vi "Extract Complementary Image ROI.vi"(8 "error in (no error)":errorcluster, 10 "Image Model":T2, 11 "ROI in":T1 {"Contours"."Type" items=["No Selection", "Point", "Line", "Rectangle", "Oval", "Polygon", "Freehand Region", "Annulus", "Unused2", "Unused3", "Broken Line", "Freehand Line", "Rotated Rectangle"]}) -> (0 "error out":errorcluster, 3 "Complementary ROI":T1 {"Contours"."Type" items=["No Selection", "Point", "Line", "Rectangle", "Oval", "Polygon", "Freehand Region", "Annulus", "Unused2", "Unused3", "Broken Line", "Freehand Line", "Rotated Rectangle"]})   [LabVIEW 2021, in "Image.lvlib"]
doc: "Builds complementary ROI."
uses:
  Image.lvlib
  <vilib>/vision/Image Controls.llb/IMAQ Image.ctl
  <vilib>/vision/NI_Vision_Development_Module.lvlib
  Error/Error.lvlib
panel:
  # "see the AlliGator License on the block diagram (Ctrl+E or Window:Show Block Diagram)"
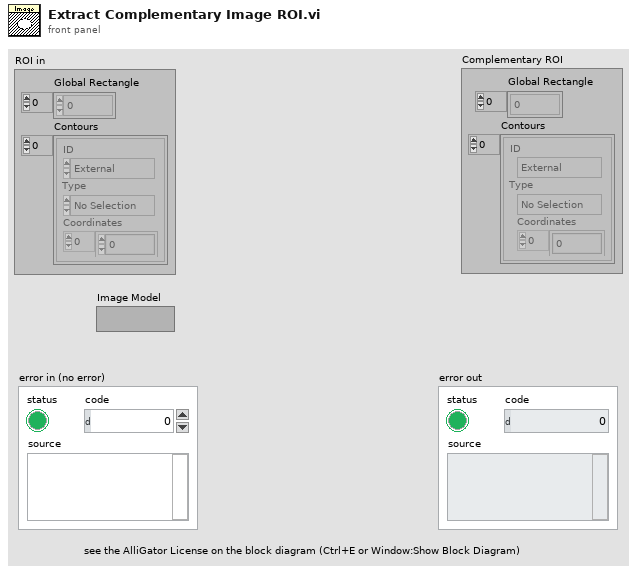
[diagram p1: front panel]
types:
  T1 = typedef "ROI Descriptor" = cluster{"Global Rectangle":i32[], "Contours":cluster{"ID":enum32{"External", "Internal"}, "Type":u32, "Coordinates":i32[]}[]}
  T2 = typedef "IMAQ Image.ctl" = refnum<image>
  T3 = typedef "Image Type" = u32
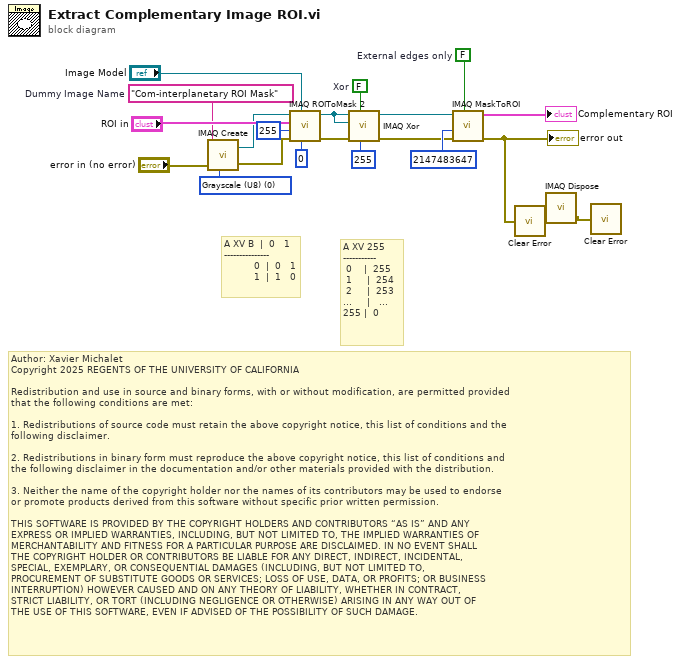
[diagram p0: block diagram]
diagram:
  w3 = FALSE  # Xor
  w11 = "Com-interplanetary ROI Mask"  # Dummy Image Name
  w12 = T3 0 items=["Grayscale (U8)", "Grayscale (I16)", "Grayscale (SGL)", "Complex (CSG)", "RGB (U32)", "HSL (U32)", "RGB (U64)", "Grayscale (U16)"] ("Image Type")
  w13 = FALSE  # External edges only
  # "Author: Xavier Michalet\nCopyright 2025 REGENTS OF THE UNIVERSITY OF CALIFORNIA\n\nRedistribution and use in source and binary forms, with or without modification, are permitted provided\nthat the following conditions are met:\n\n1. Redistributions of source code must retain the above copyright notice, this list of conditions and the\nfollowing disclaimer.\n\n2. Redistributions in binary form must reproduce the above copyright notice, this list of conditions and\nthe following disclaimer in the documentation and/or other materials provided with the distribution.\n\n3. Neither the name of the copyright holder nor the names of its contributors may be used to endorse \nor promote products derived from this software without specific prior written permission.\n\nTHIS SOFTWARE IS PROVIDED BY THE COPYRIGHT HOLDERS AND CONTRIBUTORS “AS IS” AND ANY \nEXPRESS OR IMPLIED WARRANTIES, INCLUDING, BUT NOT LIMITED TO, THE IMPLIED WARRANTIES OF\nMERCHANTABILITY AND FITNESS FOR A PARTICULAR PURPOSE ARE DISCLAIMED. IN NO EVENT SHALL\nTHE COPYRIGHT HOLDER OR CONTRIBUTORS BE LIABLE FOR ANY DIRECT, INDIRECT, INCIDENTAL, \nSPECIAL, EXEMPLARY, OR CONSEQUENTIAL DAMAGES (INCLUDING, BUT NOT LIMITED TO, \nPROCUREMENT OF SUBSTITUTE GOODS OR SERVICES; LOSS OF USE, DATA, OR PROFITS; OR BUSINESS\nINTERRUPTION) HOWEVER CAUSED AND ON ANY THEORY OF LIABILITY, WHETHER IN CONTRACT, \nSTRICT LIABILITY, OR TORT (INCLUDING NEGLIGENCE OR OTHERWISE) ARISING IN ANY WAY OUT OF\nTHE USE OF THIS SOFTWARE, EVEN IF ADVISED OF THE POSSIBILITY OF SUCH DAMAGE."
  # "A XV 255\n-----------\n 0    |  255  \n 1     |  254\n 2     |  253\n...     |   ...\n255 |  0"
  # "A XV B  |  0   1\n---------------\n          0  |  0   1\n          1  |  1   0"
  n1 = call "IMAQ Create"("Image Name"=w11, "Image Type"=w12, "error in (no error)"="error in (no error)") -> ("New Image"=w8:T2, "error out"=w9:errorcluster)  [unwired: 2 in]
  n2 = call "IMAQ ROIToMask 2"("Background Value (0)"=0, "Image Model"="Image Model", "error in (no error)"=w9, "Filling Value (255)"=255, "ROI Descriptor"="ROI in", "Image"=w8) -> ("error out"=w17:errorcluster, "Image Out"=w18:T2)  [unwired: 3 in, 1 out]
  n3 = call "IMAQ Xor"("Constant"=i64 255, "Xor/Xnor (Xor)"=w3, "error in (no error)"=w17, "Image Dst"=w18, "Image Src A"=w18) -> ("error out"=w6:errorcluster, "Image Dst Out"=w5:T2)  [unwired: 5 in]
  n4 = call "IMAQ MaskToROI"("External edges only (T)"=w13, "Image"=w5, "Max number of vectors in ROI"=2147483647, "error in (no error)"=w6) -> ("ROI Descriptor"=→"Complementary ROI":T1, "error out"=w7:errorcluster)  [unwired: 3 in, 1 out]
  "error out" <- w7
  n5 = call "Clear Error.vi"("Error In"=w7) -> ("no Error Out"=w2:errorcluster)  [unwired: 8 in]
  n6 = call "IMAQ Dispose"("error in (no error)"=w2) -> ("error out"=w1:errorcluster)  [unwired: 5 in]
  n7 = call "Clear Error.vi"("Error In"=w1) -> ()  [unwired: 8 in, 1 out]
